vi "down shift.vi"(11 "2048 2":dbl[][](array[numeric])) -> (3 "2048":dbl[][](array[numeric]))   [LabVIEW 2015]
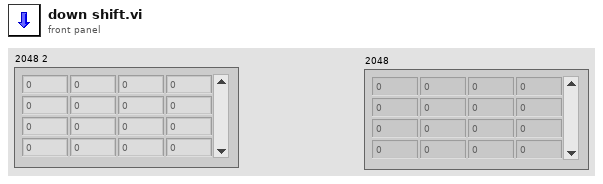
[diagram p1: front panel]
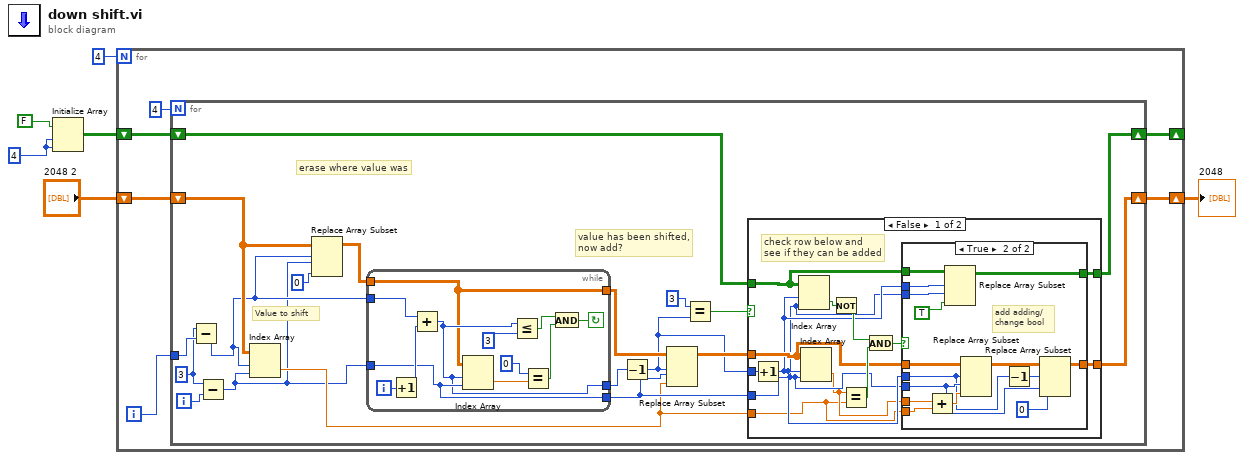
[diagram p0: block diagram]
diagram:
  w3 = 4
  n1 = Initialize Array(FALSE, w3, w3) -> (w1:bool[][])
  n2 = for {
    N: 4 -> [_]
    shift-right: [w8] -> _
    shift-left: w1 -> [w9]
    shift-right: [w7] -> w4
    shift-left: "2048 2" -> [w11]
    i -> [w10]
    n3 = for {
      N: 4 -> [_]
      tunnel: w10 -> [w17]
      shift-right: [w22] -> w8
      shift-left: w9 -> [w23]
      shift-right: [w21] -> w7
      shift-left: w11 -> [w19]
      i -> [w14]
      w15 = 3
      # "erase where value was"
      # "value has been shifted,\nnow add?"
      # "Value to shift"
      n4 = Subtract(x=w15, y=w17) -> (x-y=w16:i32)
      n5 = Subtract(x=w15, y=w14) -> (x-y=w13:i32)
      n6 = Index Array(array=w19, index (row)=w16, index (col)=w13) -> (element=w24:dbl)
      n7 = Replace Array Subset(array=w19, new element=0, index (row)=w16, index (col)=w13) -> (w20:dbl[][])
      n8 = while {
        tunnel: w16 -> [w75]
        tunnel: w13 -> [w67]
        tunnel: w20 -> [w65]
        tunnel: [w67] -> w27
        tunnel: [w66] -> w26
        tunnel: [w65] -> w31
        i -> [w74]
        stop <- w70 continue-if-true
        n9 = Increment(x=w74) -> (x+1=w71:i32)
        n10 = Add(x=w75, y=w71) -> (x+y=w66:i32)
        n11 = Index Array(array=w65, index (row)=w66, index (col)=w67) -> (element=w73:dbl)
        n12 = Less Or Equal?(x=w66, y=3) -> (x <= y?=w68:bool)
        n13 = Equal?(x=0, y=w73) -> (x = y?=w72:bool)
        n14 = And(x=w68, y=w72) -> (x .and. y?=w70:bool)
      }
      n15 = Decrement(x=w26) -> (x-1=w25:i32)
      n16 = Replace Array Subset(array=w31, new element=w24, index (row)=w25, index (col)=w27) -> (w28:dbl[][])
      n17 = Equal?(x=3, y=w25) -> (x = y?=w29:bool)
      n18 = case shown="False" w29 {
        tunnel: w28 -> [w38 w62]
        tunnel: w27 -> [w36 _]
        tunnel: w25 -> [w44 _]
        tunnel: w24 -> [w34 _]
        tunnel: w23 -> [w40 w63]
        tunnel: [w33 w63] -> w22
        tunnel: [w32 w62] -> w21
        frame False {
          # "check row below and \nsee if they can be added"
          n19 = Increment(x=w44) -> (x+1=w37:i32)
          n20 = Index Array(array=w40, index (row)=w37, index (col)=w36) -> (element=w42:bool)
          n21 = Index Array(array=w38, index (row)=w37, index (col)=w36) -> (element=w35:dbl)
          n22 = Not(x=w42) -> (.not. x?=w41:bool)
          n23 = Equal?(x=w35, y=w34) -> (x = y?=w43:bool)
          n24 = And(x=w41, y=w43) -> (x .and. y?=w39:bool)
          n25 = case shown="True" w39 {
            tunnel: w40 -> [w46 w61]
            tunnel: w36 -> [_ w60]
            tunnel: w37 -> [_ w59]
            tunnel: w38 -> [w45 w57]
            tunnel: w37 -> [_ w48]
            tunnel: w36 -> [_ w49]
            tunnel: w35 -> [_ w55]
            tunnel: w34 -> [_ w54]
            tunnel: [w46 w53] -> w33
            tunnel: [w45 w51] -> w32
            frame False {
            }
            frame True {
              # "add adding/\nchange bool"
              n26 = Add(x=w55, y=w54) -> (x+y=w56:dbl)
              n27 = Replace Array Subset(array=w61, new element=TRUE, index (row)=w59, index (col)=w60) -> (w53:bool[][])
              n28 = Replace Array Subset(array=w57, new element=w56, index (row)=w48, index (col)=w49) -> (w52:dbl[][])
              n29 = Decrement(x=w48) -> (x-1=w47:i32)
              n30 = Replace Array Subset(array=w52, new element=0, index (row)=w47, index (col)=w49) -> (w51:dbl[][])
            }
          }
        }
        frame True {
          # "if it is row 3 then,\n no adds to check"
        }
      }
    }
  }
  "2048" <- w4
